vi "Get_Rise_Fall_Time.vi"(0 "dt":dbl, 5 "Transition_Points":i32[](array[numeric])) -> (4 "Rise_Time (s)":dbl, 6 "Fall_Time (s)":dbl)   [LabVIEW 2021]
doc: "This VI Get the rise and fall time when transition points and dt were given in."
uses:
  <vilib>/gmath/NI_Gmath.lvlib
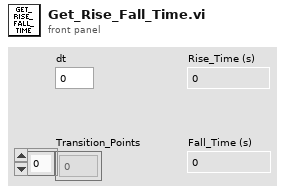
[diagram p1: front panel]
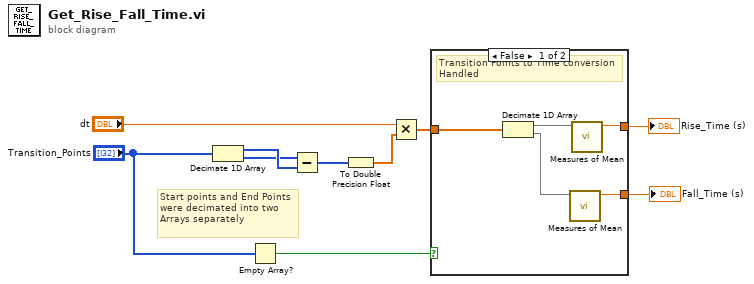
[diagram p0: block diagram]
diagram:
  # "Start points and End Points were decimated into two Arrays separately"
  n1 = Decimate 1D Array("Transition_Points") -> (w4:i32[], w3:i32[])
  n2 = Empty Array?(array="Transition_Points") -> (empty?=w7:bool)
  n3 = Subtract(x=w3, y=w4) -> (x-y=w6:i32[])
  n4 = To Double Precision Float(number=w6) -> (double precision float=w5:dbl[])
  n5 = Multiply(x="dt", y=w5) -> (x*y=w1:dbl[])
  n6 = case shown="False" w7 {
    tunnel: [w15 _] -> w10
    tunnel: [w14 _] -> w9
    tunnel: w1 -> [w13 _]
    frame False {
      # "Transition Points to Time conversion Handled"
      n7 = Decimate 1D Array(w13) -> (w12:dbl[], w11:dbl[])
      n8 = call <vilib>:"Measures of Mean.vi"("x array"=w11) -> ("mean value"=w15:dbl)  [unwired: 9 in, 1 out]
      n9 = call <vilib>:"Measures of Mean.vi"("x array"=w12) -> ("mean value"=w14:dbl)  [unwired: 9 in, 1 out]
    }
    frame True {
      # "No transition Points Condition handled"
    }
  }
  "Rise_Time (s)" <- w9
  "Fall_Time (s)" <- w10
